vi "GetGrowInfo.vi"(0 "XRef":T7, 1 "State In":T6) -> (14 "Grow Info":T2, 15 "Fatal Error Out":T1)   [LabVIEW 2015, in "Get Object Parameters.xnode"]
uses:
  Get Object Parameters.xnode
  <vilib>/XNodeSupport/XNodeXNodeRef.ctl
  State.ctl
  <vilib>/XNodeSupport/XNodeGrowInfo.ctl
  <vilib>/XNodeSupport/XNodeBounds.ctl
  <vilib>/XNodeSupport/XNodeInt.ctl
  <vilib>/XNodeSupport/XNodeBool.ctl
  <vilib>/XNodeSupport/XNodeErrorCluster.ctl
  dimensions.vi
  <vilib>/XNodeSupport/NI_XNodeSupport.lvlib
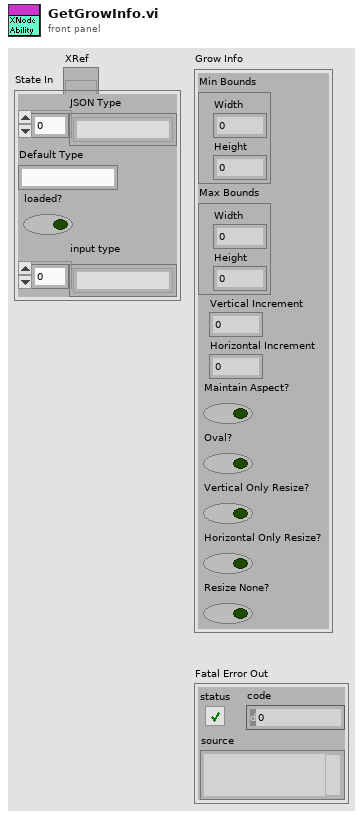
[diagram p1: front panel]
types:
  T1 = typedef "NI_XNodeSupport.lvlib/XNodeErrorCluster.ctl" = errorcluster
  T2 = typedef "NI_XNodeSupport.lvlib/XNodeGrowInfo.ctl" = cluster{"Min Bounds":T3, "Max Bounds":T3, "Vertical Increment":T4, "Horizontal Increment":T4, "Maintain Aspect?":T5, "Oval?":T5, "Vertical Only Resize?":T5, "Horizontal Only Resize?":T5, "Resize None?":T5}
  T3 = typedef "NI_XNodeSupport.lvlib/XNodeBounds.ctl" = cluster{"Width":T4, "Height":T4}
  T4 = typedef "NI_XNodeSupport.lvlib/XNodeInt.ctl" = i32
  T5 = typedef "NI_XNodeSupport.lvlib/XNodeBool.ctl" = bool
  T6 = typedef "Get Object Parameters.xnode/State.ctl" = cluster{"JSON Type":string[], "Default Type":string, "loaded?":bool, "input type":string[]}
  T7 = typedef "NI_XNodeSupport.lvlib/XNodeXNodeRef.ctl" = refnum<vi>
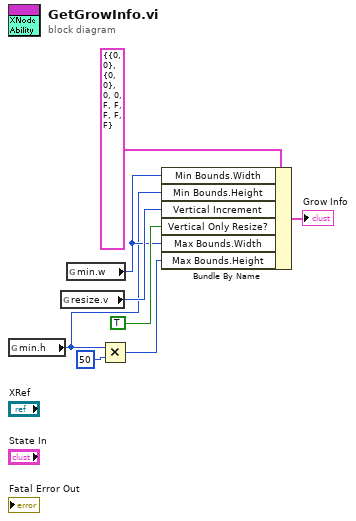
[diagram p0: block diagram]
diagram:
  n1 = global read "dimensions.vi" "min.h"() -> (w3:i32)
  n2 = global read "dimensions.vi" "resize.v"() -> (w6:i32)
  n3 = global read "dimensions.vi" "min.w"() -> (w4:i32)
  n4 = Multiply(x=w3, y=50) -> (x*y=w1:i32)
  n5 = Bundle By Name(cluster=T2 {"Min Bounds"={"Width"=0, "Height"=0}, "Max Bounds"={"Width"=0, "Height"=0}, "Vertical Increment"=0, "Horizontal Increment"=0, "Maintain Aspect?"=FALSE, "Oval?"=FALSE, "Vertical Only Resize?"=FALSE, "Horizontal Only Resize?"=FALSE, "Resize None?"=FALSE} ("Grow Info"), "Min Bounds.Width"=w4, "Min Bounds.Height"=w3, "Vertical Increment"=w6, "Vertical Only Resize?"=T5 TRUE, "Max Bounds.Width"=w4, "Max Bounds.Height"=w1) -> (→"Grow Info":T2)
